vi "SetBinning.vi"(8 "error in (no error)":errorcluster, 9 "Setting.Binning.BinY":i32, 10 "Setting.Binning.BinX":i32, 11 "Camera_Prime95B in":refnum<class "Camera_Prime95B.lvclass">) -> (0 "error out":errorcluster, 3 "Camera_Prime95B out":refnum<class "Camera_Prime95B.lvclass">)   [LabVIEW 2020, in "Camera_Prime95B.lvlib" / "Camera_Prime95B.lvclass"]
uses:
  Camera_Prime95B.lvclass
  Camera_Prime95B.lvclass/Camera_Prime95B.ctl
  E:/Development/DevHardSoftware/MMicroscopyAF/Model/Real Hardware/Camera_Prime95B/Camera_Prime95B/Dependencies/PVCamNET.dll
  Dependencies/PVCamNET.dll
  HAL Layer/Component/Camera/Camera/Camera.lvclass
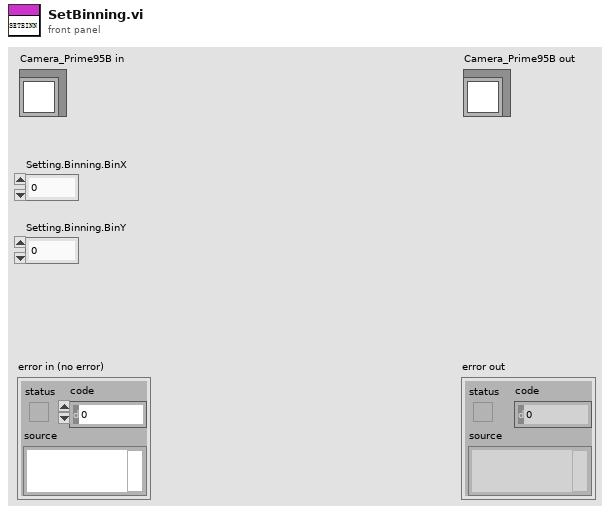
[diagram p1: front panel]
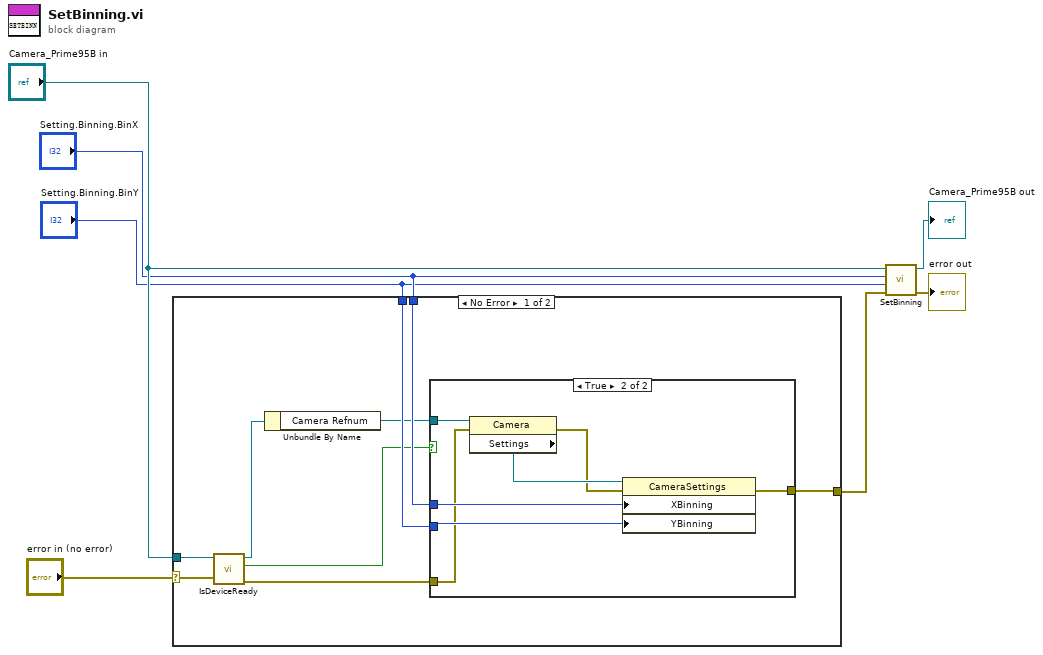
[diagram p0: block diagram]
diagram:
  n1 = case shown="No Error" "error in (no error)" {
    selector: "error in (no error)" -> [w13 w25]
    tunnel: [w14 w25] -> w4
    tunnel: "Camera_Prime95B in" -> [w12 _]
    tunnel: "Setting.Binning.BinX" -> [w16 _]
    tunnel: "Setting.Binning.BinY" -> [w15 _]
    frame No Error {
      n2 = call-dynamic "IsDeviceReady.vi"("error in (no error)"=w13, "Camera_Prime95B in"=w12) -> ("error out"=w10:errorcluster, "Ready?"=w11:bool, "Camera_Prime95B out"=w9:refnum<class "Camera_Prime95B.lvclass">)  [unwired: 7 in]
      n3 = Unbundle By Name(w9) -> ("Camera Refnum"=w8:refnum<k24>)
      n4 = case shown="True" w11 {
        tunnel: [w17 w24] -> w14
        tunnel: w8 -> [_ w21]
        tunnel: w16 -> [_ w20]
        tunnel: w15 -> [_ w19]
        tunnel: w10 -> [w17 w18]
        frame False {
        }
        frame True {
          n5 = property class="Camera"(reference=w21, error in=w18) -> (error out=w22:errorcluster, "Settings"=w23:refnum<k24>)  [unwired: 1 out]
          n6 = property class="CameraSettings"(reference=w23, error in=w22, "XBinning"=w20, "YBinning"=w19) -> (error out=w24:errorcluster)  [unwired: 1 out]
        }
      }
    }
    frame Error {
    }
  }
  n7 = call-parent "SetBinning.vi"("error in (no error)"=w4, "Setting.Binning.BinY"="Setting.Binning.BinY", "Setting.Binning.BinX"="Setting.Binning.BinX", "Camera in"="Camera_Prime95B in") -> ("error out"=→"error out":errorcluster, "Camera out"=→"Camera_Prime95B out":refnum<class "Camera_Prime95B.lvclass">)  [unwired: 6 in]
